vi "PCert-Application-Dir-Support.vi"(8 "error in":errorcluster, 11 "Support Resource Relative Filepath":string) -> (0 "error out":errorcluster, 3 "Support Path":path)   [LabVIEW 2013]
panel:
  out "appended path":path
  out "Deploy Root":path
  out "Provider Root":path
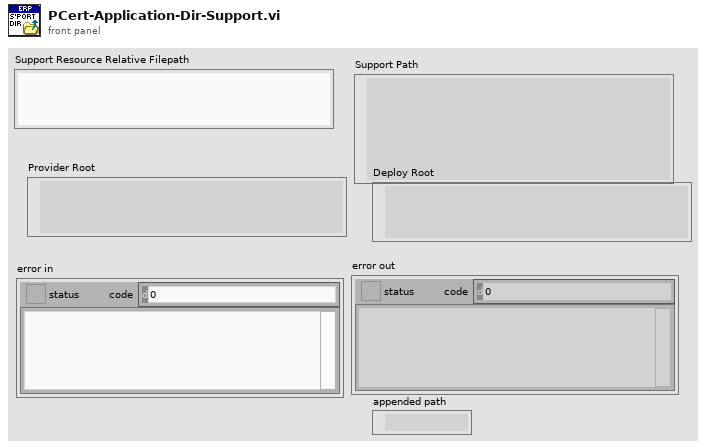
[diagram p1: front panel]
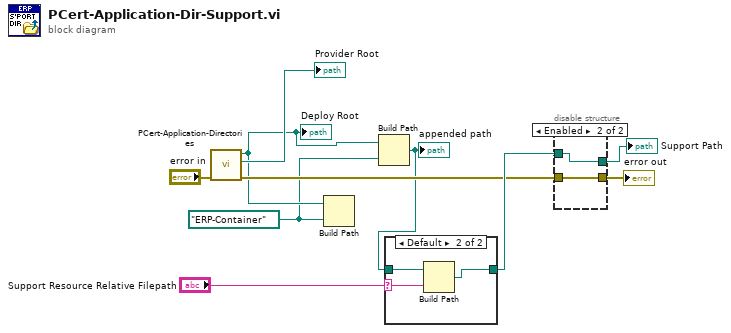
[diagram p0: block diagram]
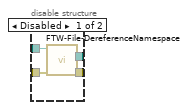
[diagram p2: hidden frame]
diagram:
  w2 = path "ERP-Container"
  n1 = call "PCert-Application-Directories.vi"("error in"="error in") -> ("error out"=w8:errorcluster, "Provider Root"=→"Provider Root":path, "Deploy Root"=w3:path)  [unwired: 8 in]
  "Deploy Root" <- w3
  n2 = Build Path(base path=w3, name or relative path=w2) -> ()  [unwired: 1 out]
  n3 = Build Path(base path=w3, name or relative path=w2) -> (appended path=w1:path)
  "appended path" <- w1
  n4 = case shown="Default" "Support Resource Relative Filepath" {
    selector: "Support Resource Relative Filepath" -> [_ w12]
    tunnel: [w11 w14] -> w9
    tunnel: w1 -> [w11 w13]
    frame "" {
    }
    frame Default {
      n5 = Build Path(base path=w13, name or relative path=w12) -> (appended path=w14:path)
    }
  }
  n6 = disable-structure shown="Enabled" {
    disable-tunnel: w9 -> [w18 w19]
    disable-tunnel: w8 -> [w17 w20]
    disable-tunnel: [w16 w19] -> w7
    disable-tunnel: [w15 w20] -> w6
    frame Disabled {
      n7 = call "FTW-File-DereferenceNamespace.vi"("error in"=w17, "Base Filepath"=w18) -> ("error out"=w15:errorcluster, "Actual Filepath"=w16:path)  [unwired: 8 in]
    }
    frame Enabled {
    }
  }
  "Support Path" <- w7
  "error out" <- w6
